vi "LibXML_EditXMLTree.vi"(6 "mode":T3(ring), 8 "error in":errorcluster, 9 "XML-tree":T1[](array[typedef]), 10 "node":u32, 11 "doc":u32) -> (0 "error out":errorcluster, 1 "first written node":u32, 2 "node copy out":u32, 3 "doc copy out":u32)   [LabVIEW 2019, in "Tools.lvlib" / "LibXML.lvlib"]
doc: "There are 4 edit-modes:\n1. Remove the node from the document\n2. Insert the XML-tree into the document as a child of the selected node\n3. Insert the XML-tree into the document as a sybling of the selected node\n4. Replace the selected node by the XML-tree in the document."
uses:
  LibXML.lvlib
  LibXML_Element.ctl
  LibXML_Attribute.ctl
panel:
  # "This software is FREE licensed under the GNU Lesser General Public License (see license.txt)."
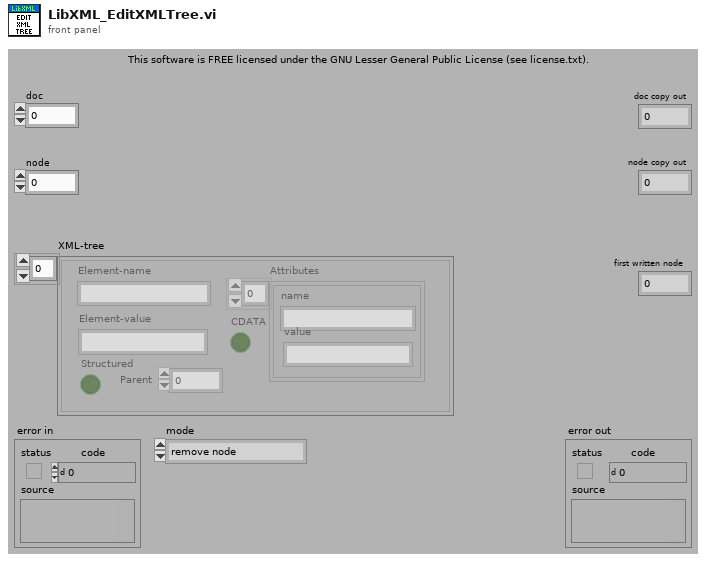
[diagram p1: front panel]
types:
  T1 = typedef "Tools.lvlib/LibXML.lvlib/LibXML_Element.ctl" = cluster{"Element-name":string, "Attributes":T2[], "Element-value":string, "CDATA":bool, "Parent":i32, "Structured":bool}
  T2 = typedef "Tools.lvlib/LibXML.lvlib/LibXML_Attribute.ctl" = cluster{"name":string, "value":string}
  T3 = enum16{"remove node", "replace node", "insert node after", "add new childnode"}
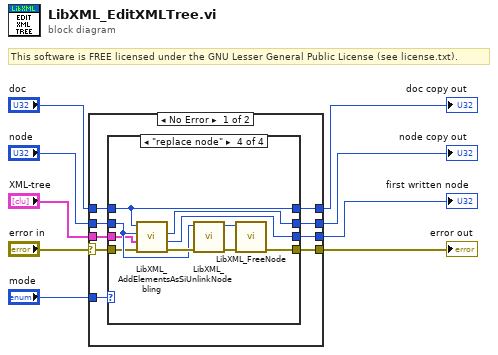
[diagram p0: block diagram]
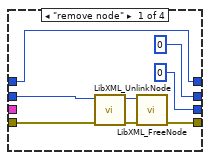
[diagram p2: hidden frame]
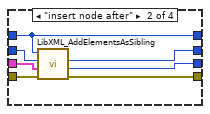
[diagram p3: hidden frame]
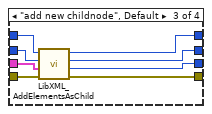
[diagram p4: hidden frame]
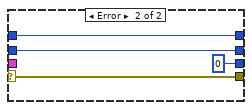
[diagram p5: hidden frame]
diagram:
  # "This software is FREE licensed under the GNU Lesser General Public License (see license.txt)."
  n1 = case shown="No Error" "error in" {
    selector: "error in" -> [w18 w55]
    tunnel: [w16 w55] -> w9
    tunnel: "doc" -> [w17 w54]
    tunnel: "node" -> [w15 w53]
    tunnel: [w14 w54] -> w5
    tunnel: [w13 w53] -> w4
    tunnel: [w12 u32 0 ("first written node")] -> w3
    tunnel: "XML-tree" -> [w11 _]
    tunnel: "mode" -> [w10 _]
    frame No Error {
      n2 = case shown="\"replace node\"" w10 {
        tunnel: w18 -> [w22 w33 w41 w42]
        tunnel: [w23 w32 w40 w51] -> w16
        tunnel: w11 -> [_ w31 w39 w43]
        tunnel: w17 -> [w26 w29 w38 w45]
        tunnel: w15 -> [w21 w30 w37 w44]
        tunnel: [w26 w29 w36 w45] -> w14
        tunnel: [u32 0 ("parent copy out") w27 w35 w46] -> w13
        tunnel: [u32 0 ("parent copy out") w28 w34 w47] -> w12
        frame "remove node" {
          n3 = call "LibXML_UnlinkNode.vi"("error in"=w22, "node"=w21) -> ("error out"=w25:errorcluster, "node copy out"=w24:u32)  [unwired: 8 in]
          n4 = call "LibXML_FreeNode.vi"("error in"=w25, "node"=w24) -> ("error out"=w23:errorcluster)  [unwired: 9 in]
        }
        frame "insert node after" {
          n5 = call "LibXML_AddElementsAsSibling.vi"("error in"=w33, "XML-tree"=w31, "node in"=w30, "doc"=w29) -> ("error out"=w32:errorcluster, "first written node"=w28:u32, "Node-out"=w27:u32)  [unwired: 4 in, 1 out]
        }
        frame "add new childnode", Default {
          n6 = call "LibXML_AddElementsAsChild.vi"("error in"=w41, "XML-tree"=w39, "parent"=w37, "doc"=w38) -> ("error out"=w40:errorcluster, "first written node"=w34:u32, "parent copy out"=w35:u32, "doc copy out"=w36:u32)  [unwired: 4 in]
        }
        frame "replace node" {
          n7 = call "LibXML_AddElementsAsSibling.vi"("error in"=w42, "XML-tree"=w43, "node in"=w44, "doc"=w45) -> ("error out"=w48:errorcluster, "first written node"=w47:u32, "Node-out"=w46:u32)  [unwired: 4 in, 1 out]
          n8 = call "LibXML_UnlinkNode.vi"("error in"=w48, "node"=w44) -> ("error out"=w50:errorcluster, "node copy out"=w49:u32)  [unwired: 8 in]
          n9 = call "LibXML_FreeNode.vi"("error in"=w50, "node"=w49) -> ("error out"=w51:errorcluster)  [unwired: 9 in]
        }
      }
    }
    frame Error {
    }
  }
  "error out" <- w9
  "doc copy out" <- w5
  "node copy out" <- w4
  "first written node" <- w3
